vi "LSCI332 GetGenPar.vi"(8 "error in (no error)":errorcluster, 9 "Input":u32(ring) caption="Entrée de\nTempérature" items=["A", "B"], 10 "Parameter":T1=enum."All", 11 "VISA Rsrc":refnum<visa-resource-name>="GPIB0::12::INSTR") -> (0 "error out":errorcluster, 1 "Filter Points":u16, 2 "Filtering":bool, 3 "Curve Number":u32, 4 "Window %":u16, 5 "Compensation":bool, 7 "Sensor Type":T2(ring))   [LabVIEW 2019]
doc: "Ce VI envoie la commande Zone? au contrôlleur, ce qui retourne les paramètres de la zone spécifiée."
uses:
  <userlib>/LSCI 332 V2/InputPars.ctl
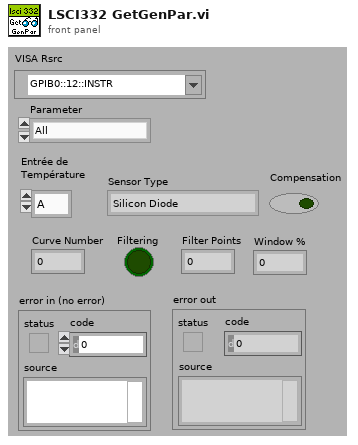
[diagram p1: front panel]
types:
  T1 = typedef "InputPars.ctl" = enum16{"Input Type", "Filter", "Input Curve", "All"}
  T2 = enum16{"Silicon Diode", "GaAlAs", "100 Ohms Platinum/250", "100 Ohms Platinum/500", "1000 Ohms Platinum", "NTC RTD", "Thermocouple 25mv", "Thermocouple 50mv", "2.5V 1mA", "7.5V 1mA"}
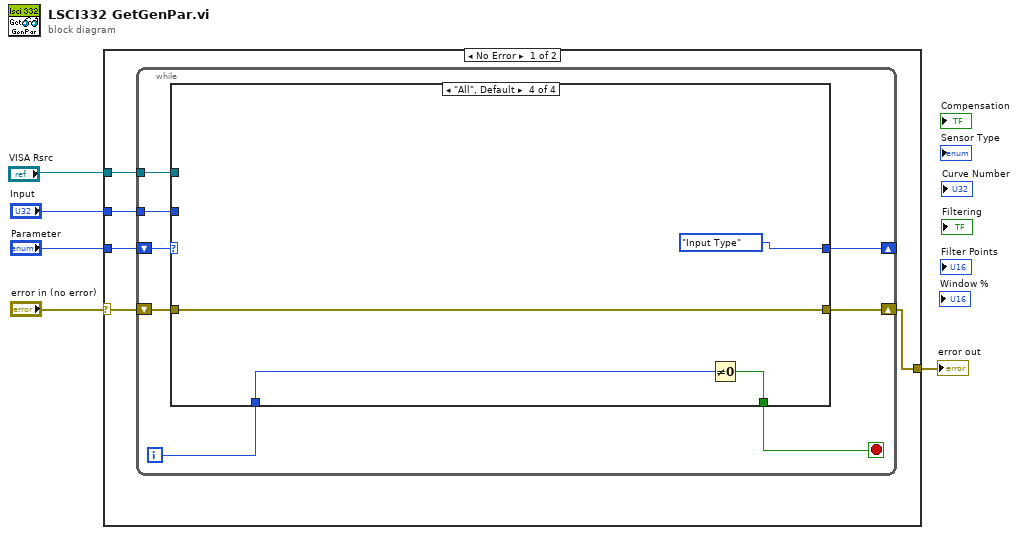
[diagram p0: block diagram]
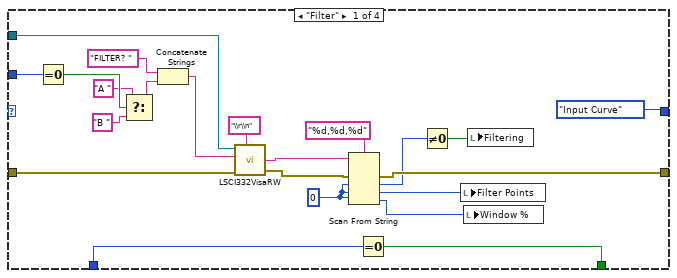
[diagram p2: hidden frame]
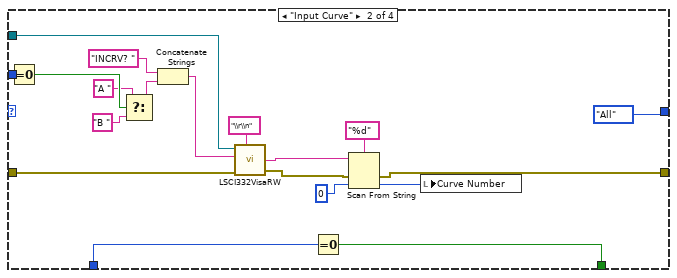
[diagram p3: hidden frame]
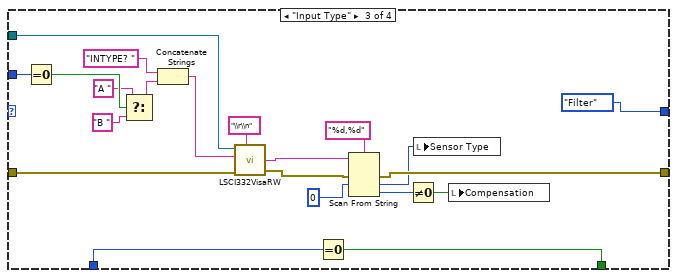
[diagram p4: hidden frame]
diagram:
  n1 = case shown="No Error" "error in (no error)" {
    selector: "error in (no error)" -> [w9 w85]
    tunnel: "VISA Rsrc" -> [w10 _]
    tunnel: [w8 w85] -> w4
    tunnel: "Input" -> [w7 _]
    tunnel: "Parameter" -> [w6 _]
    frame No Error {
      n2 = while {
        tunnel: w10 -> [w18]
        tunnel: w7 -> [w15]
        shift-right: [w16] -> w8
        shift-left: w9 -> [w17]
        shift-right: [w11] -> _
        shift-left: w6 -> [w14]
        i -> [w12]
        stop <- w13 stop-if-true
        n3 = case shown="\"All\", Default" w14 {
          tunnel: w18 -> [w39 w58 w79 _]
          tunnel: w17 -> [w38 w57 w78 w84]
          tunnel: [w32 w51 w72 w84] -> w16
          tunnel: w15 -> [w31 w50 w67 _]
          tunnel: [w20 w42 w61 w83] -> w13
          tunnel: w12 -> [w21 w43 w62 w82]
          tunnel: [InputPars."Input Curve" ("Parameter") InputPars."All" ("Parameter") InputPars."Filter" ("Parameter") InputPars."Input Type" ("Parameter")] -> w11
          frame "Filter" {
            w22 = u16 0
            n4 = Equal To 0?(x=w31) -> (x = 0?=w30:bool)
            n5 = Select(t="A " ("string"), s=w30, f="B " ("string")) -> (s? t:f=w27:string)
            n6 = Concatenate Strings("FILTER? " ("string"), w27) -> (w36:string)
            n7 = call <userlib>:"LSCI332VisaRW.vi"("error in (no error)"=w38, "EOS (Aucun)"="\\r\\n", "ChaineCom"=w36, "VISA Rsrc"=w39) -> ("error out"=w33:errorcluster, "ChaineRep"=w35:string)  [unwired: 3 in, 2 out]
            n8 = Scan From String(format string="%d,%d,%d" ("regular expression"), input string=w35, error in=w33, default 1=w22, default 2=w22, default 3=w22) -> (error out=w32:errorcluster, output 1=w26:u16, output 2=w24:u16, output 3=w23:u16)  [unwired: 1 in, 2 out]
            n9 = Equal To 0?(x=w21) -> (x = 0?=w20:bool)
            n10 = Not Equal To 0?(x=w26) -> (x != 0?=w25:bool)
            n11 = local write "Filter Points"(w24) -> ()
            n12 = local write "Window %"(w23) -> ()
            n13 = local write "Filtering"(w25) -> ()
          }
          frame "Input Curve" {
            n14 = Equal To 0?(x=w50) -> (x = 0?=w49:bool)
            n15 = Select(t="A " ("string"), s=w49, f="B " ("string")) -> (s? t:f=w46:string)
            n16 = Concatenate Strings("INCRV? " ("string"), w46) -> (w55:string)
            n17 = call <userlib>:"LSCI332VisaRW.vi"("error in (no error)"=w57, "EOS (Aucun)"="\\r\\n", "ChaineCom"=w55, "VISA Rsrc"=w58) -> ("error out"=w52:errorcluster, "ChaineRep"=w54:string)  [unwired: 3 in, 2 out]
            n18 = Equal To 0?(x=w43) -> (x = 0?=w42:bool)
            n19 = Scan From String(format string="%d" ("regular expression"), input string=w54, error in=w52, default 1=u32 0 ("Curve Number")) -> (error out=w51:errorcluster, output 1=w45:u32)  [unwired: 1 in, 2 out]
            n20 = local write "Curve Number"(w45) -> ()
          }
          frame "Input Type" {
            n21 = Equal To 0?(x=w67) -> (x = 0?=w66:bool)
            n22 = Select(t="A " ("string"), s=w66, f="B " ("string")) -> (s? t:f=w63:string)
            n23 = Concatenate Strings("INTYPE? " ("string"), w63) -> (w76:string)
            n24 = call <userlib>:"LSCI332VisaRW.vi"("error in (no error)"=w78, "EOS (Aucun)"="\\r\\n", "ChaineCom"=w76, "VISA Rsrc"=w79) -> ("error out"=w73:errorcluster, "ChaineRep"=w75:string)  [unwired: 3 in, 2 out]
            n25 = Equal To 0?(x=w62) -> (x = 0?=w61:bool)
            n26 = Scan From String(format string="%d,%d" ("regular expression"), input string=w75, error in=w73, default 1=u16 0) -> (error out=w72:errorcluster, output 1=w69:u16, output 2=w71:i32)  [unwired: 2 in, 2 out]
            n27 = Not Equal To 0?(x=w71) -> (x != 0?=w68:bool)
            n28 = local write "Sensor Type"(w69) -> ()
            n29 = local write "Compensation"(w68) -> ()
          }
          frame "All", Default {
            n30 = Not Equal To 0?(x=w82) -> (x != 0?=w83:bool)
          }
        }
      }
    }
    frame Error {
    }
  }
  "error out" <- w4
